vi "Status.Builder.Get State Pointer.vi"(11 "Builder Status in":refnum<class "Status.Builder.lvclass">) -> (2 "Builder State Pointer":refnum<class "DSF.Engine.Pointer.Status.Builder.State.lvclass">, 3 "Builder Status out":refnum<class "Status.Builder.lvclass">)   [LabVIEW 2016, in "DSF.Engine.lvlib" / "Status.Builder.lvclass"]
uses:
  Status.Builder.lvclass
  Pointer/DSF.Engine.Pointer.Status.Builder.State.lvclass
  Status.Builder.lvclass/Status.Builder.ctl
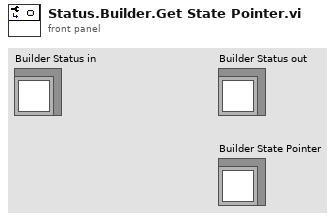
[diagram p1: front panel]
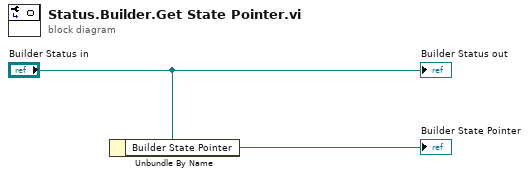
[diagram p0: block diagram]
diagram:
  n1 = Unbundle By Name("Builder Status in") -> ("Builder State Pointer"=→"Builder State Pointer":refnum<class "DSF.Engine.Pointer.Status.Builder.State.lvclass">)
  "Builder Status out" <- "Builder Status in"
